vi "TestComplete.vi"(7 "Socket":i32, 8 "error in (no error)":errorcluster, 9 "SerialNumber":string, 10 "TestResult":string, 11 "SignalProcessing in":refnum<class "SignalProcessing.lvclass">) -> (0 "error out":errorcluster, 3 "SignalProcessing out":refnum<class "SignalProcessing.lvclass">)   [LabVIEW 2019, in "SignalProcessing.lvlib" / "SignalProcessing.lvclass"]
uses:
  SignalProcessing.lvclass
  SignalProcessing Global.vi
  <resource>/objmgr/ni.dex.rc
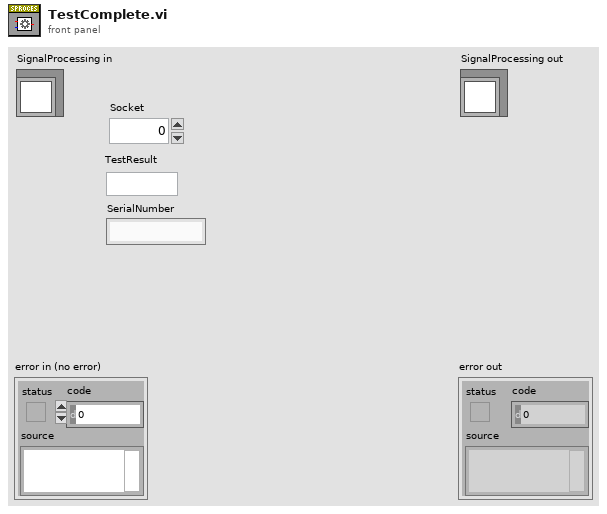
[diagram p1: front panel]
types:
  T1 = cluster{"Socket":i32, "SerialNumber":string, "TestResult":string}
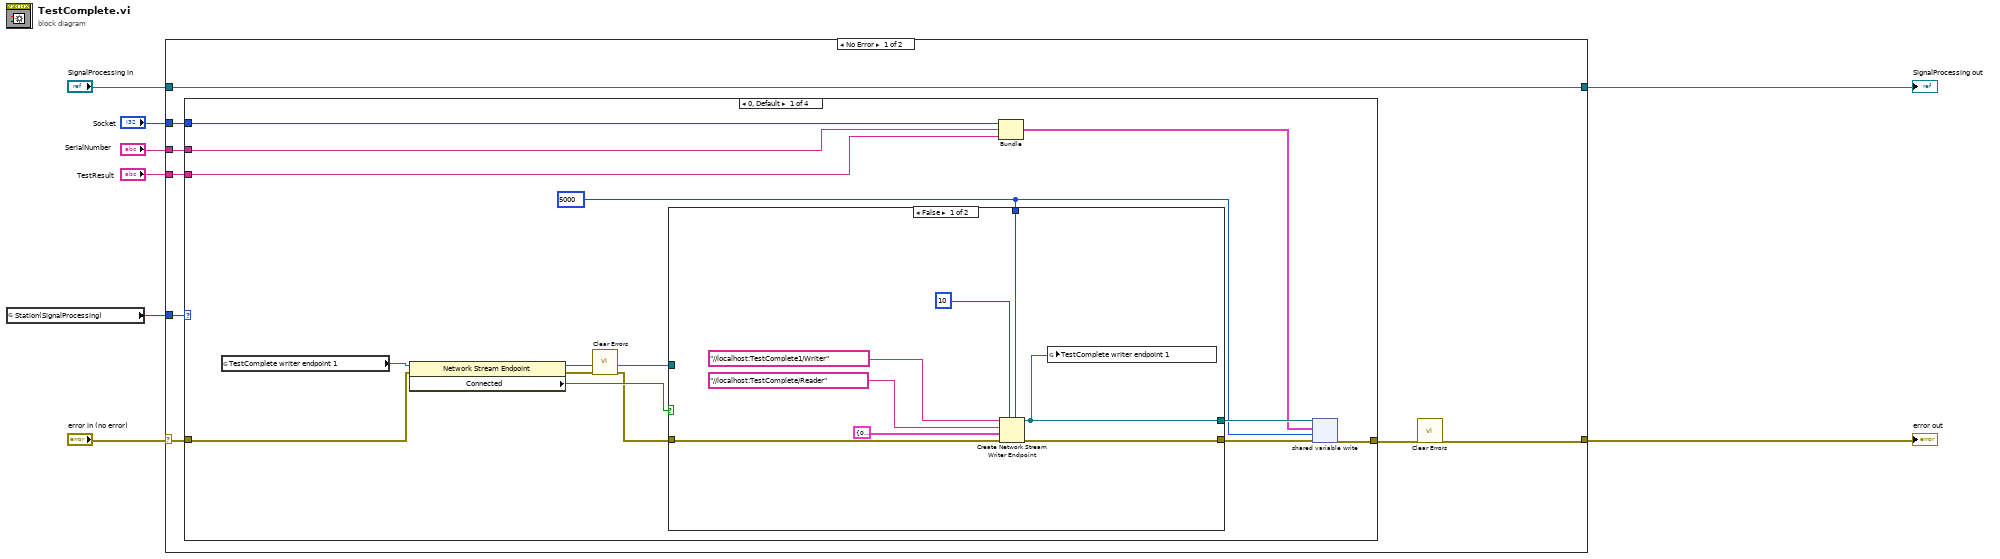
[diagram p0: block diagram]
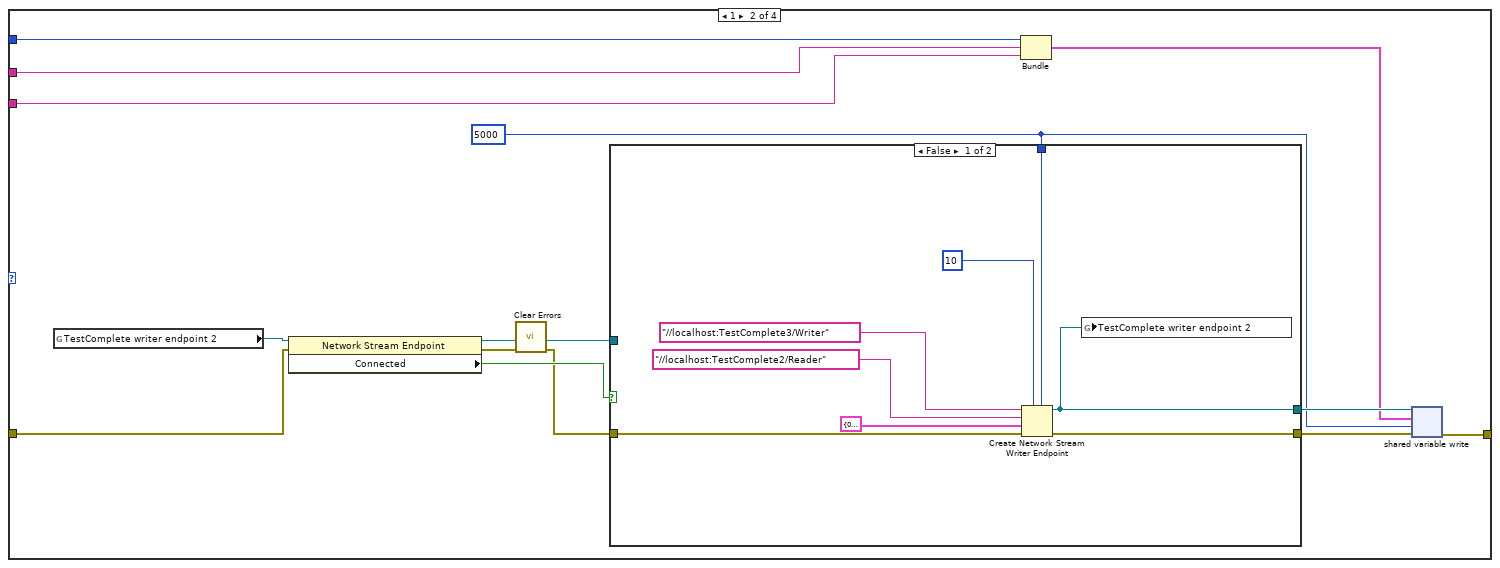
[diagram p3: hidden frame]
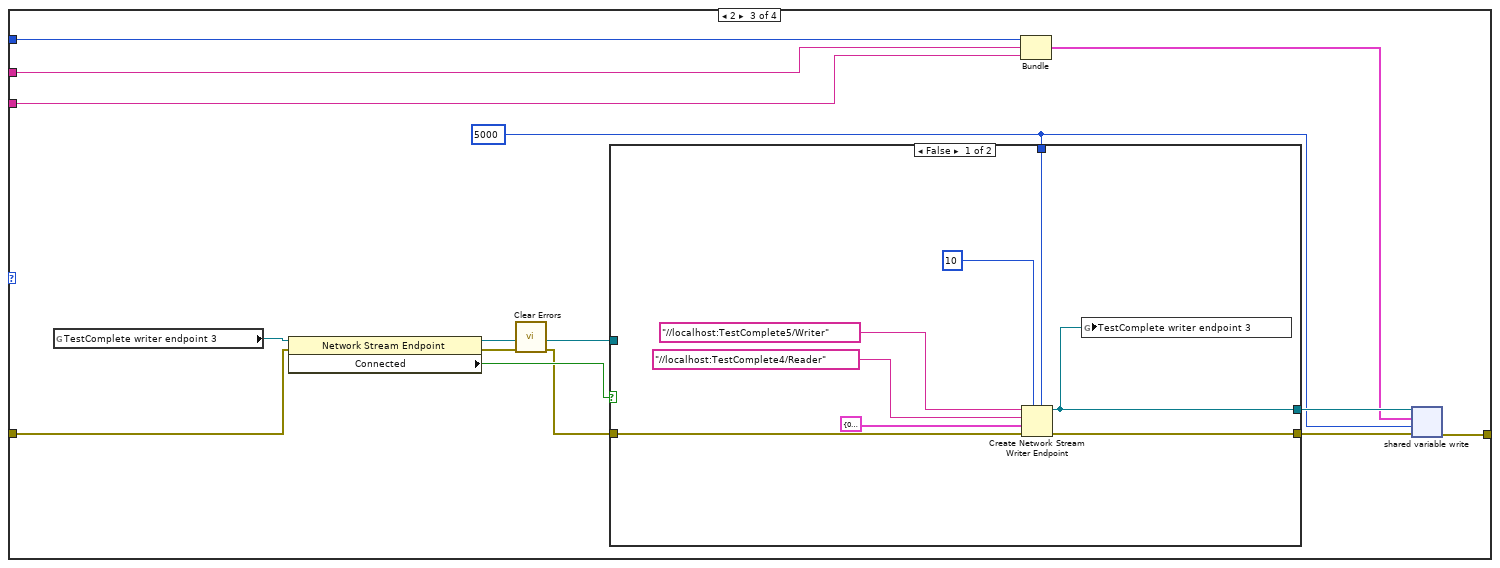
[diagram p5: hidden frame]
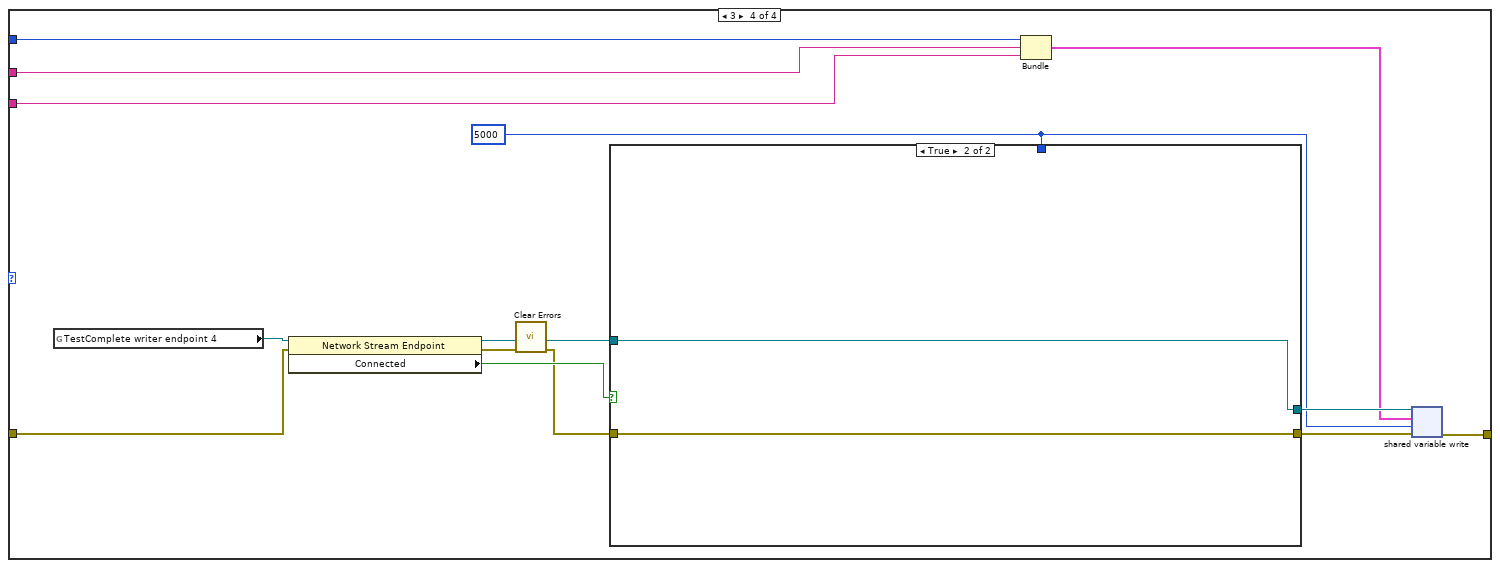
[diagram p7: hidden frame]
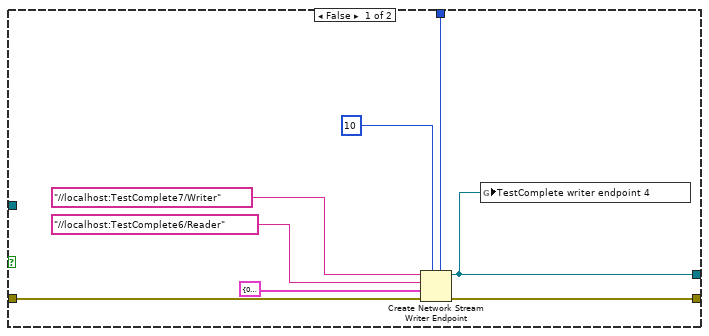
[diagram p8: hidden frame]
diagram:
  n1 = global read "SignalProcessing Global.vi" "Station(SignalProcessing)"() -> (w1:i32)
  n2 = case shown="No Error" "error in (no error)" {
    selector: "error in (no error)" -> [w10 w114]
    tunnel: [w11 w114] -> w7
    tunnel: [w16 w113] -> w5
    tunnel: "SignalProcessing in" -> [w16 w113]
    tunnel: "TestResult" -> [w13 _]
    tunnel: "Socket" -> [w15 _]
    tunnel: "SerialNumber" -> [w14 _]
    tunnel: w1 -> [w9 _]
    frame No Error {
      n3 = case shown="0, Default" w9 {
        tunnel: w15 -> [w30 w54 w78 w102]
        tunnel: w14 -> [w29 w53 w77 w101]
        tunnel: w13 -> [w28 w52 w76 w100]
        tunnel: [w24 w48 w72 w96] -> w12
        tunnel: w10 -> [w19 w43 w67 w91]
        frame 0, Default {
          w17 = 5000 ("timeout in ms (-1)")
          n4 = global read "SignalProcessing Global.vi" "TestComplete writer endpoint 1"() -> (w18:refnum<k21>)
          n5 = property class="Network Stream Endpoint"(reference=w18, error in=w19) -> (reference out=w20:refnum<k21>, error out=w23:errorcluster, "Connected"=w22:bool)
          n6 = call <vilib>:"Clear Errors.vi"("error in (no error)"=w23) -> ("error out"=w21:errorcluster)  [unwired: 5 in, 1 out]
          n7 = case shown="False" w22 {
            tunnel: w21 -> [w38 w39]
            tunnel: [w37 w39] -> w27
            tunnel: [w32 w40] -> w26
            tunnel: w20 -> [_ w40]
            tunnel: w17 -> [w31 _]
            frame False {
              n8 = Create Network Stream Writer Endpoint(5:w31, 7:10 ("writer buffer size"), 8:w38, 9:T1 {"Socket"=0, "SerialNumber"="", "TestResult"=""}, 10:"//localhost:TestComplete/Reader" ("reader name"), 11:"//localhost:TestComplete1/Writer" ("reader name")) -> (0:w37:errorcluster, 3:w32:refnum<k21>)  [unwired: 1 in]
              n9 = global write "SignalProcessing Global.vi" "TestComplete writer endpoint 1"(w32) -> ()
            }
            frame True {
            }
          }
          n10 = Bundle("Socket"=w30, "SerialNumber"=w29, "TestResult"=w28) -> (w25:T1)  [unwired: 1 in]
          n11 = shared-variable-write(w26, w27, w25, w17) -> (w24:errorcluster)  [unwired: 2 out]
        }
        frame 1 {
          w41 = 5000 ("timeout in ms (-1)")
          n12 = global read "SignalProcessing Global.vi" "TestComplete writer endpoint 2"() -> (w42:refnum<k21>)
          n13 = property class="Network Stream Endpoint"(reference=w42, error in=w43) -> (reference out=w44:refnum<k21>, error out=w47:errorcluster, "Connected"=w46:bool)
          n14 = call <vilib>:"Clear Errors.vi"("error in (no error)"=w47) -> ("error out"=w45:errorcluster)  [unwired: 5 in, 1 out]
          n15 = case shown="False" w46 {
            tunnel: w45 -> [w62 w63]
            tunnel: [w61 w63] -> w51
            tunnel: [w56 w64] -> w50
            tunnel: w44 -> [_ w64]
            tunnel: w41 -> [w55 _]
            frame False {
              n16 = Create Network Stream Writer Endpoint(5:w55, 7:10 ("writer buffer size"), 8:w62, 9:T1 {"Socket"=0, "SerialNumber"="", "TestResult"=""}, 10:"//localhost:TestComplete2/Reader" ("reader name"), 11:"//localhost:TestComplete3/Writer" ("reader name")) -> (0:w61:errorcluster, 3:w56:refnum<k21>)  [unwired: 1 in]
              n17 = global write "SignalProcessing Global.vi" "TestComplete writer endpoint 2"(w56) -> ()
            }
            frame True {
            }
          }
          n18 = Bundle("Socket"=w54, "SerialNumber"=w53, "TestResult"=w52) -> (w49:T1)  [unwired: 1 in]
          n19 = shared-variable-write(w50, w51, w49, w41) -> (w48:errorcluster)  [unwired: 2 out]
        }
        frame 2 {
          w65 = 5000 ("timeout in ms (-1)")
          n20 = global read "SignalProcessing Global.vi" "TestComplete writer endpoint 3"() -> (w66:refnum<k21>)
          n21 = property class="Network Stream Endpoint"(reference=w66, error in=w67) -> (reference out=w68:refnum<k21>, error out=w71:errorcluster, "Connected"=w70:bool)
          n22 = call <vilib>:"Clear Errors.vi"("error in (no error)"=w71) -> ("error out"=w69:errorcluster)  [unwired: 5 in, 1 out]
          n23 = case shown="False" w70 {
            tunnel: w69 -> [w86 w87]
            tunnel: [w85 w87] -> w75
            tunnel: [w80 w88] -> w74
            tunnel: w68 -> [_ w88]
            tunnel: w65 -> [w79 _]
            frame False {
              n24 = Create Network Stream Writer Endpoint(5:w79, 7:10 ("writer buffer size"), 8:w86, 9:T1 {"Socket"=0, "SerialNumber"="", "TestResult"=""}, 10:"//localhost:TestComplete4/Reader" ("reader name"), 11:"//localhost:TestComplete5/Writer" ("reader name")) -> (0:w85:errorcluster, 3:w80:refnum<k21>)  [unwired: 1 in]
              n25 = global write "SignalProcessing Global.vi" "TestComplete writer endpoint 3"(w80) -> ()
            }
            frame True {
            }
          }
          n26 = Bundle("Socket"=w78, "SerialNumber"=w77, "TestResult"=w76) -> (w73:T1)  [unwired: 1 in]
          n27 = shared-variable-write(w74, w75, w73, w65) -> (w72:errorcluster)  [unwired: 2 out]
        }
        frame 3 {
          w89 = 5000 ("timeout in ms (-1)")
          n28 = global read "SignalProcessing Global.vi" "TestComplete writer endpoint 4"() -> (w90:refnum<k21>)
          n29 = property class="Network Stream Endpoint"(reference=w90, error in=w91) -> (reference out=w92:refnum<k21>, error out=w95:errorcluster, "Connected"=w94:bool)
          n30 = call <vilib>:"Clear Errors.vi"("error in (no error)"=w95) -> ("error out"=w93:errorcluster)  [unwired: 5 in, 1 out]
          n31 = case shown="True" w94 {
            tunnel: w93 -> [w110 w111]
            tunnel: [w109 w111] -> w99
            tunnel: [w104 w112] -> w98
            tunnel: w92 -> [_ w112]
            tunnel: w89 -> [w103 _]
            frame False {
              n32 = Create Network Stream Writer Endpoint(5:w103, 7:10 ("writer buffer size"), 8:w110, 9:T1 {"Socket"=0, "SerialNumber"="", "TestResult"=""}, 10:"//localhost:TestComplete6/Reader" ("reader name"), 11:"//localhost:TestComplete7/Writer" ("reader name")) -> (0:w109:errorcluster, 3:w104:refnum<k21>)  [unwired: 1 in]
              n33 = global write "SignalProcessing Global.vi" "TestComplete writer endpoint 4"(w104) -> ()
            }
            frame True {
            }
          }
          n34 = Bundle("Socket"=w102, "SerialNumber"=w101, "TestResult"=w100) -> (w97:T1)  [unwired: 1 in]
          n35 = shared-variable-write(w98, w99, w97, w89) -> (w96:errorcluster)  [unwired: 2 out]
        }
      }
      n36 = call <vilib>:"Clear Errors.vi"("error in (no error)"=w12) -> ("error out"=w11:errorcluster)  [unwired: 5 in, 1 out]
    }
    frame Error {
    }
  }
  "error out" <- w7
  "SignalProcessing out" <- w5
